vi "YJoint_Test.vi"() -> ()   [LabVIEW 2018]
uses:
  cluster_enum.ctl
  <vilib>/Utility/error.llb/DialogType.ctl
  <vilib>/DAQmx/read.llb/DAQmx Read (Analog 1D Wfm NChan NSamp).vi
  <vilib>/Waveform/WDTOps.llb/WDT Get Waveform Time Array DBL.vi
  <vilib>/DAQmx/configure/timing.llb/DAQmx Timing (Sample Clock).vi
  <vilib>/DAQmx/miscellaneous.llb/DAQmx Fill In Error Info.vi
  <resource>/objmgr/daqmx.rc
panel:
  out "Accel Card":waveform(dbl)[](graph) caption="Waveform Chart"
  in  "Tab Control":enum32{"Telemetry", "DAQ Settings"}(tab)
  in  "Accel Tare":bool caption="Reset"
  in  "Strain Card 1 Tare":bool caption="Reset"
  in  "Stop 4":bool caption="Stop"
  out "Save Path":path caption="Path"
  in  "Test Name":string caption="String"
  in  "Save 2":bool caption="Save"
  out "Accel Card Rate":dbl caption="Numeric"
  in  "Accel Card Sample Rate Setpoint":dbl=100.0 caption="Numeric"
  in  "Accel Card 1 Samples Per Loop":i32=100 caption="Numeric"
  in  "Strain Card 1 Rate Setpoint":dbl=1000.0 caption="Numeric"
  out "Strain Card 1 Rate":dbl caption="Numeric"
  in  "Strain Card 1 Samples Per Loop":i32=100 caption="Numeric"
  out "Strain Card 1":waveform(dbl)[](graph) caption="Waveform Chart"
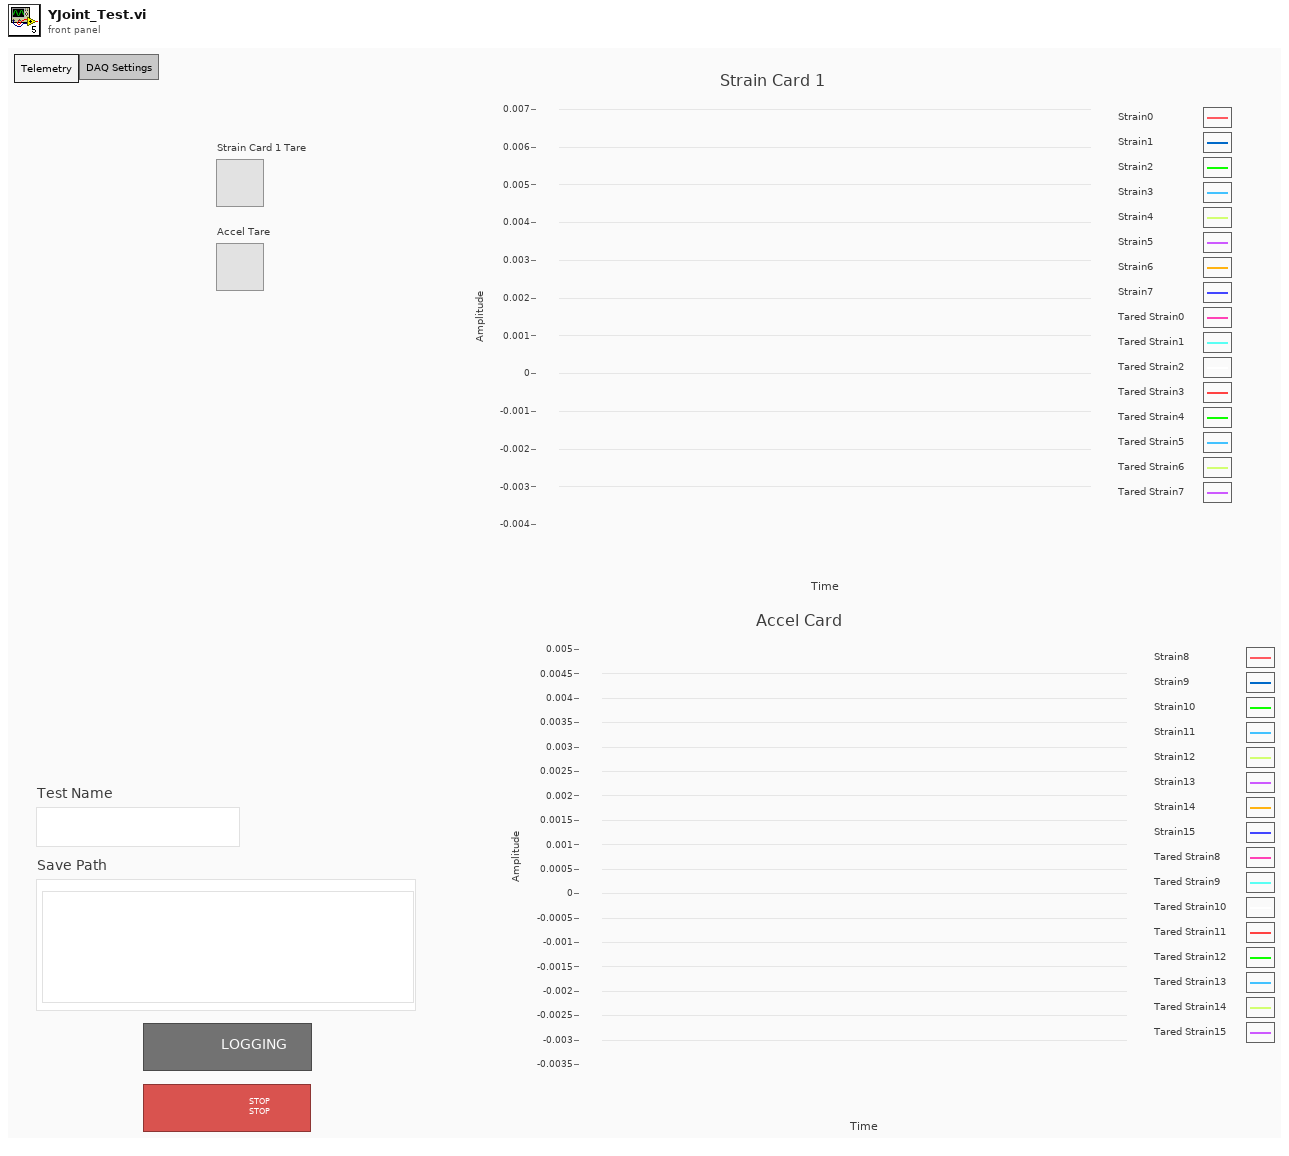
[diagram p1: front panel]
types:
  T1 = typedef "DialogType.ctl" = u16
  T2 = enum16{"open", "open or create", "create or replace", "create", "open (read-only)"}
  T3 = typedef "cluster_enum.ctl" = enum16{"Strain Card 2", "Strain Card 2 Tared", "Strain Card 1 Tared", "Strain Card 1", "Accel Card 1", "Accel Card 1 Tared", ""}
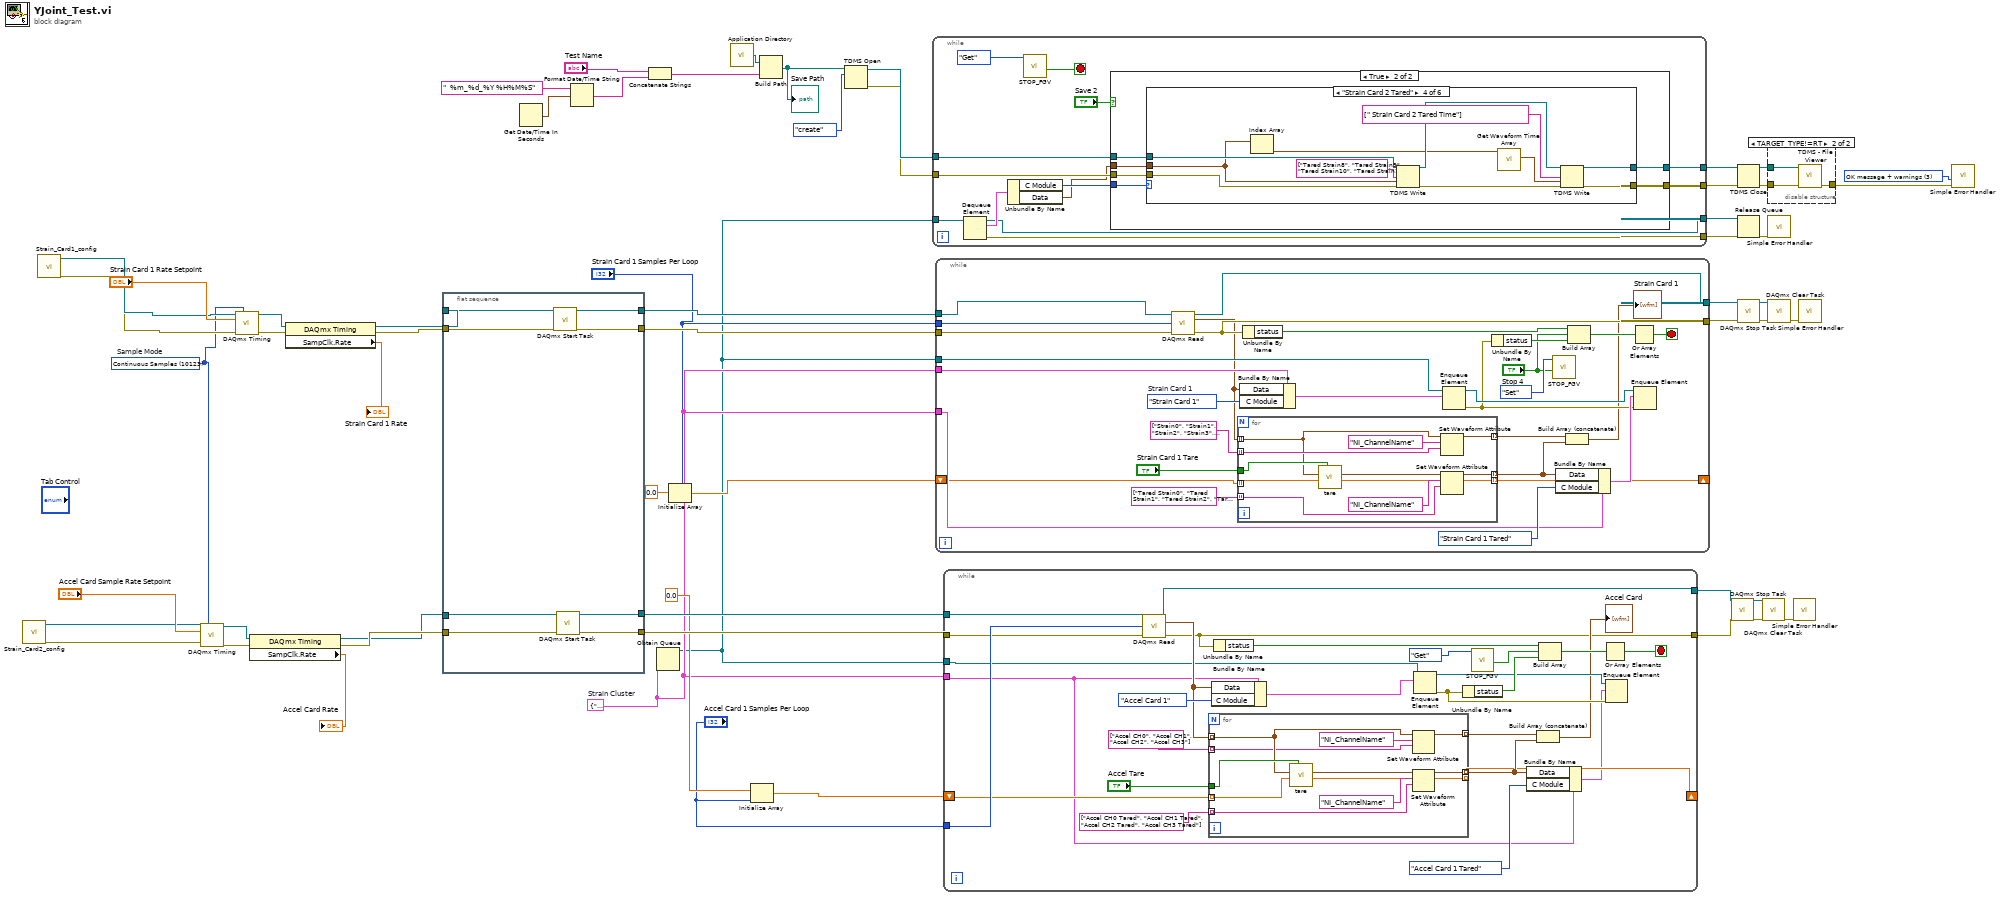
[diagram p0: block diagram]
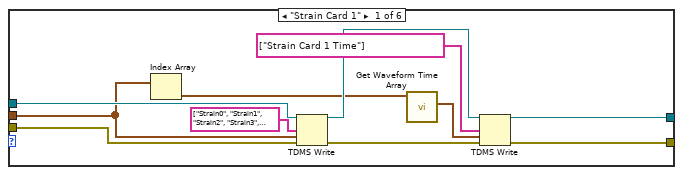
[diagram p4: hidden frame]
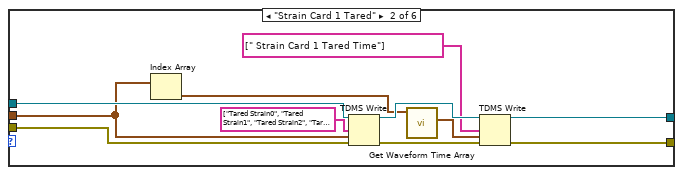
[diagram p5: hidden frame]
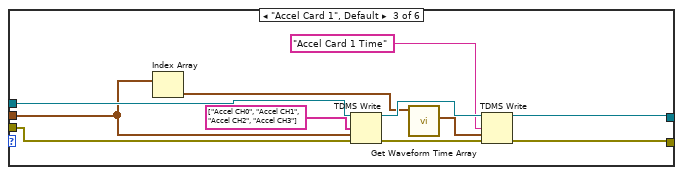
[diagram p6: hidden frame]
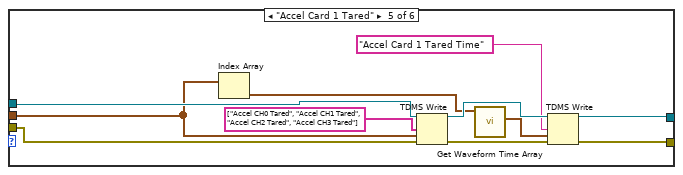
[diagram p7: hidden frame]
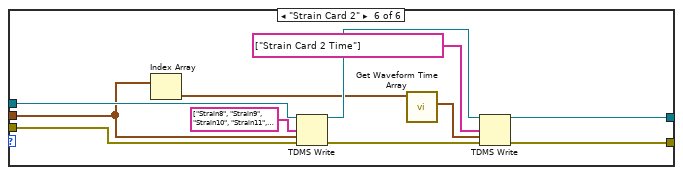
[diagram p8: hidden frame]
diagram:
  w35 = T1 3 items=["no dialog", "OK message", "continue or stop message", "OK message + warnings", "continue/stop + warnings"] ("type of dialog (OK msg:1)")
  w8 = cluster{"C Module":T3, " Data":waveform(dbl)[]} {"C Module"=enum."Strain Card 2", " Data"=[]}  # Strain Cluster
  w1 = 10123 items=["Finite Samples"=10178, "Continuous Samples"=10123, "Hardware Timed Single Point"=12522]  # Sample Mode
  n1 = call "Strain_Card2_config.vi"() -> ("error out"=w16:errorcluster, "task out"=w17:refnum<k21>)  [unwired: 10 in]
  n2 = call "Strain_Card1_config.vi"() -> ("error out"=w22:errorcluster, "task out"=w23:refnum<k21>)  [unwired: 10 in]
  n3 = call-poly <vilib>:"DAQmx Timing.vi"("task/channels in"=w17, "sample mode"=w1, "rate"="Accel Card Sample Rate Setpoint", "error in"=w16) -> ("task out"=w21:refnum<k21>, "error out"=w20:errorcluster)  [unwired: 10 in]
  n4 = call-poly <vilib>:"DAQmx Timing.vi"("task/channels in"=w23, "sample mode"=w1, "rate"="Strain Card 1 Rate Setpoint", "error in"=w22) -> ("task out"=w58:refnum<k21>, "error out"=w57:errorcluster)  [unwired: 10 in]
  n5 = property class="DAQmx Timing"(reference=w21, error in=w20) -> (reference out=w14:refnum<k21>, error out=w15:errorcluster, "SampClk.Rate"=→"Accel Card Rate":dbl)
  n6 = property class="DAQmx Timing"(reference=w58, error in=w57) -> (reference out=w56:refnum<k21>, error out=w55:errorcluster, "SampClk.Rate"=→"Strain Card 1 Rate":dbl)
  n7 = flat-sequence {
    tunnel: [w66] -> w52
    tunnel: w56 -> [w65]
    tunnel: w55 -> [w64]
    tunnel: [w63] -> w51
    tunnel: w15 -> [w62]
    tunnel: w14 -> [w61]
    tunnel: [w60] -> w13
    tunnel: [w59] -> w12
    frame #0 {
      n8 = call <vilib>:"DAQmx Start Task.vi"("task/channels in"=w65, "error in"=w64) -> ("task out"=w66:refnum<k21>, "error out"=w63:errorcluster)  [unwired: 12 in]
      n9 = call <vilib>:"DAQmx Start Task.vi"("task/channels in"=w61, "error in"=w62) -> ("task out"=w60:refnum<k21>, "error out"=w59:errorcluster)  [unwired: 12 in]
    }
  }
  n10 = Get Date/Time In Seconds() -> (seconds since 1Jan1904=w44:timestamp)
  n11 = Format Date/Time String(time format string (%c)="  %m_%d_%Y %H%M%S", seconds (now)=w44) -> (date/time string=w41:string)  [unwired: 1 in]
  n12 = Concatenate Strings("Test Name", w41) -> (w40:string)
  n13 = Obtain Queue(element data type=w8) -> (queue out=w7:refnum<queue>)  [unwired: 4 in, 2 out]
  n14 = Initialize Array(0.0 ("element"), "Strain Card 1 Samples Per Loop") -> (w24:dbl[])
  n15 = call <vilib>:"Application Directory.vi"() -> ("Application Directory"=w42:path)
  n16 = Initialize Array(0.0 ("element"), "Accel Card 1 Samples Per Loop") -> (w9:dbl[])
  n17 = Build Path(base path=w42, name or relative path=w40) -> (appended path=w39:path)
  "Save Path" <- w39
  n18 = TDMS Open(10:T2."create" ("operation"), 11:w39) -> (0:w36:errorcluster, 3:w37:refnum<k34>)  [unwired: 5 in]
  n19 = while {
    tunnel: w7 -> [w79]
    tunnel: w37 -> [w76]
    tunnel: w36 -> [w75]
    tunnel: [w73] -> w31
    tunnel: [w72] -> w30
    tunnel: [w68] -> w28
    tunnel: [w67] -> w27
    stop <- w70 stop-if-true
    n20 = Dequeue Element(queue=w79) -> (queue out=w68:refnum<queue>, element=w78:cluster{"C Module":T3, " Data":waveform(dbl)[]}, error out=w67:errorcluster)  [unwired: 2 in, 1 out]
    n21 = Unbundle By Name(w78) -> ("C Module"=w77:T3, "Data"=w74:waveform(dbl)[])
    n22 = call "STOP_FGV.vi"("Mode"=enum16{"Set", "Get"}."Get") -> ("Get Value"=w70:bool)  [unwired: 9 in, 1 out]
    n23 = case shown="True" "Save 2" {
      tunnel: w77 -> [_ w87]
      tunnel: w76 -> [w81 w86]
      tunnel: w75 -> [w80 w85]
      tunnel: w74 -> [_ w84]
      tunnel: [w81 w83] -> w73
      tunnel: [w80 w82] -> w72
      frame False {
      }
      frame True {
        n24 = case shown="\"Strain Card 2 Tared\"" w87 {
          tunnel: w86 -> [w98 w109 w114 w131 w135 w153]
          tunnel: w85 -> [w97 w108 w113 w130 w136 w152]
          tunnel: w84 -> [w91 w102 w112 w124 w134 w146]
          tunnel: [w93 w104 w111 w126 w138 w148] -> w83
          tunnel: [w94 w105 w110 w127 w137 w149] -> w82
          frame "Strain Card 1" {
            n25 = Index Array(array=w91) -> (element=w90:waveform(dbl))  [unwired: 1 in]
            n26 = TDMS Write(0:w98, 7:string[] ["Strain0", "Strain1", "Strain2", "Strain3", "Strain4", "Strain5", "Strain6", "Strain7"] ("channel name(s) in (Untitled)"), 9:w91, 11:w97) -> (4:w96:refnum<k34>, 15:w95:errorcluster)  [unwired: 2 in, 2 out]
            n27 = call-poly <vilib>:"Get Waveform Time Array.vi"("waveform in"=w90) -> ("X array"=w89:timestamp[])  [unwired: 9 in, 1 out]
            n28 = TDMS Write(0:w96, 7:string[] ["Strain Card 1 Time"] ("channel name(s) in (Untitled)"), 9:w89, 11:w95) -> (4:w93:refnum<k34>, 15:w94:errorcluster)  [unwired: 2 in, 2 out]
          }
          frame "Strain Card 1 Tared" {
            n29 = Index Array(array=w102) -> (element=w101:waveform(dbl))  [unwired: 1 in]
            n30 = TDMS Write(0:w109, 7:string[] ["Tared Strain0", "Tared Strain1", "Tared Strain2", "Tared Strain3", "Tared Strain4", "Tared Strain5", "Tared Strain6", "Tared Strain7"] ("channel name(s) in (Untitled)"), 9:w102, 11:w108) -> (4:w107:refnum<k34>, 15:w106:errorcluster)  [unwired: 2 in, 2 out]
            n31 = call-poly <vilib>:"Get Waveform Time Array.vi"("waveform in"=w101) -> ("X array"=w100:timestamp[])  [unwired: 9 in, 1 out]
            n32 = TDMS Write(0:w107, 7:string[] [" Strain Card 1 Tared Time"] ("channel name(s) in (Untitled)"), 9:w100, 11:w106) -> (4:w104:refnum<k34>, 15:w105:errorcluster)  [unwired: 2 in, 2 out]
          }
          frame "Accel Card 1", Default {
            n33 = Index Array(array=w112) -> (element=w118:waveform(dbl))  [unwired: 1 in]
            n34 = TDMS Write(0:w114, 7:string[] ["Accel CH0", "Accel CH1", "Accel CH2", "Accel CH3"] ("channel name(s) in (Untitled)"), 9:w112, 11:w113) -> (4:w120:refnum<k34>, 15:w119:errorcluster)  [unwired: 2 in, 2 out]
            n35 = call-poly <vilib>:"Get Waveform Time Array.vi"("waveform in"=w118) -> ("X array"=w117:timestamp[])  [unwired: 9 in, 1 out]
            n36 = TDMS Write(0:w120, 7:"Accel Card 1 Time", 9:w117, 11:w119) -> (4:w111:refnum<k34>, 15:w110:errorcluster)  [unwired: 2 in, 2 out]
          }
          frame "Strain Card 2 Tared" {
            n37 = Index Array(array=w124) -> (element=w123:waveform(dbl))  [unwired: 1 in]
            n38 = TDMS Write(0:w131, 7:string[] ["Tared Strain8", "Tared Strain9", "Tared Strain10", "Tared Strain11", "Tared Strain12", "Tared Strain13", "Tared Strain14", "Tared Strain15"] ("channel name(s) in (Untitled)"), 9:w124, 11:w130) -> (4:w129:refnum<k34>, 15:w128:errorcluster)  [unwired: 2 in, 2 out]
            n39 = call-poly <vilib>:"Get Waveform Time Array.vi"("waveform in"=w123) -> ("X array"=w122:timestamp[])  [unwired: 9 in, 1 out]
            n40 = TDMS Write(0:w129, 7:string[] [" Strain Card 2 Tared Time"] ("channel name(s) in (Untitled)"), 9:w122, 11:w128) -> (4:w126:refnum<k34>, 15:w127:errorcluster)  [unwired: 2 in, 2 out]
          }
          frame "Accel Card 1 Tared" {
            n41 = Index Array(array=w134) -> (element=w140:waveform(dbl))  [unwired: 1 in]
            n42 = TDMS Write(0:w135, 7:string[] ["Accel CH0 Tared", "Accel CH1 Tared", "Accel CH2 Tared", "Accel CH3 Tared"] ("channel name(s) in (Untitled)"), 9:w134, 11:w136) -> (4:w142:refnum<k34>, 15:w141:errorcluster)  [unwired: 2 in, 2 out]
            n43 = call-poly <vilib>:"Get Waveform Time Array.vi"("waveform in"=w140) -> ("X array"=w139:timestamp[])  [unwired: 9 in, 1 out]
            n44 = TDMS Write(0:w142, 7:"Accel Card 1 Tared Time", 9:w139, 11:w141) -> (4:w138:refnum<k34>, 15:w137:errorcluster)  [unwired: 2 in, 2 out]
          }
          frame "Strain Card 2" {
            n45 = Index Array(array=w146) -> (element=w145:waveform(dbl))  [unwired: 1 in]
            n46 = TDMS Write(0:w153, 7:string[] ["Strain8", "Strain9", "Strain10", "Strain11", "Strain12", "Strain13", "Strain14", "Strain15"] ("channel name(s) in (Untitled)"), 9:w146, 11:w152) -> (4:w151:refnum<k34>, 15:w150:errorcluster)  [unwired: 2 in, 2 out]
            n47 = call-poly <vilib>:"Get Waveform Time Array.vi"("waveform in"=w145) -> ("X array"=w144:timestamp[])  [unwired: 9 in, 1 out]
            n48 = TDMS Write(0:w151, 7:string[] ["Strain Card 2 Time"] ("channel name(s) in (Untitled)"), 9:w144, 11:w150) -> (4:w148:refnum<k34>, 15:w149:errorcluster)  [unwired: 2 in, 2 out]
          }
        }
      }
    }
  }
  n49 = while {
    tunnel: w52 -> [w178]
    tunnel: [w182] -> w48
    tunnel: w51 -> [w177]
    tunnel: [w175] -> w47
    tunnel: w7 -> [w171]
    tunnel: w8 -> [w174]
    tunnel: w8 -> [w168]
    tunnel: "Strain Card 1 Samples Per Loop" -> [w156]
    shift-right: [w154] -> _
    shift-left: w24 -> [w155]
    stop <- w181 stop-if-true
    w173 = cluster_enum."Strain Card 1"  # Strain Card 1
    n50 = call-poly <vilib>:"DAQmx Read.vi"("task/channels in"=w178, "number of samples per channel"=w156, "error in"=w177) -> ("task out"=w182:refnum<k21>, "data"=w161:waveform(dbl)[], "error out"=w175:errorcluster)  [unwired: 10 in]
    n51 = for {
      tunnel: w161 -> [w190] mode=indexing
      tunnel: [w185] -> w162 mode=indexing
      tunnel: "Strain Card 1 Tare" -> [w193]
      tunnel: string[] ["Strain0", "Strain1", "Strain2", "Strain3", "Strain4", "Strain5", "Strain6", "Strain7"] ("channel name(s) in (Untitled)") -> [w191] mode=indexing
      tunnel: [w189] -> w158 mode=indexing
      tunnel: string[] ["Tared Strain0", "Tared Strain1", "Tared Strain2", "Tared Strain3", "Tared Strain4", "Tared Strain5", "Tared Strain6", "Tared Strain7"] ("channel name(s) in (Untitled)") -> [w186] mode=indexing
      tunnel: w155 -> [w184] mode=indexing
      tunnel: [w183] -> w154 mode=indexing
      n52 = call "tare.vi"("Tare Control"=w193, "Shift Registor"=w184, "Input Waveform"=w190) -> ("Shift Registor Out"=w183:dbl, "output waveform"=w188:waveform(dbl))  [unwired: 7 in]
      n53 = Set Waveform Attribute(5:w191, 6:"NI_ChannelName" ("name"), 7:w190) -> (3:w189:waveform(dbl))  [unwired: 1 in, 2 out]
      n54 = Set Waveform Attribute(5:w186, 6:"NI_ChannelName" ("name"), 7:w188) -> (3:w185:waveform(dbl))  [unwired: 1 in, 2 out]
    }
    n55 = Bundle By Name(cluster=w174, "Data"=w161, "C Module"=w173) -> (w172:cluster{"C Module":T3, " Data":waveform(dbl)[]})
    n56 = Unbundle By Name(w175) -> ("status"=w180:bool)
    n57 = Enqueue Element(queue=w171, element=w172) -> (queue out=w166:refnum<queue>, error out=w165:errorcluster)  [unwired: 2 in, 1 out]
    n58 = Unbundle By Name(w165) -> ("status"=w176:bool)
    n59 = call "STOP_FGV.vi"("Set Value"="Stop 4", "Mode"=enum16{"Set", "Get"}."Set") -> ()  [unwired: 8 in, 2 out]
    n60 = Bundle By Name(cluster=w168, "Data"=w162, "C Module"=cluster_enum."Strain Card 1 Tared" ("Strain Card 1")) -> (w167:cluster{"C Module":T3, " Data":waveform(dbl)[]})
    n61 = Build Array (concatenate)(w158, w162) -> (→"Strain Card 1":waveform(dbl)[])
    n62 = Build Array(w180, "Stop 4", w176) -> (w179:bool[])
    n63 = Or Array Elements(Boolean array=w179) -> (logical OR=w181:bool)
    n64 = Enqueue Element(queue=w166, element=w167, error in (no error)=w165) -> ()  [unwired: 1 in, 3 out]
  }
  n65 = while {
    tunnel: w13 -> [w205]
    tunnel: w12 -> [w203]
    tunnel: "Accel Card 1 Samples Per Loop" -> [w204]
    shift-right: [w198] -> _
    shift-left: w9 -> [w202]
    tunnel: w8 -> [w197]
    tunnel: w7 -> [w201]
    tunnel: [w200] -> w3
    tunnel: [w199] -> w2
    stop <- w196 stop-if-true
    n66 = call-poly <vilib>:"DAQmx Read.vi"("task/channels in"=w205, "number of samples per channel"=w204, "error in"=w203) -> ("task out"=w200:refnum<k21>, "data"=w210:waveform(dbl)[], "error out"=w199:errorcluster)  [unwired: 10 in]
    n67 = for {
      tunnel: w210 -> [w228] mode=indexing
      tunnel: [w231] -> w209 mode=indexing
      tunnel: "Accel Tare" -> [w232]
      tunnel: string[] ["Accel CH0 Tared", "Accel CH1 Tared", "Accel CH2 Tared", "Accel CH3 Tared"] ("channel name(s) in (Untitled)") -> [w226] mode=indexing
      tunnel: string[] ["Accel CH0", "Accel CH1", "Accel CH2", "Accel CH3"] ("channel name(s) in (Untitled)") -> [w225] mode=indexing
      tunnel: [w227] -> w206 mode=indexing
      tunnel: [w223] -> w198 mode=indexing
      tunnel: w202 -> [w222] mode=indexing
      n68 = call "tare.vi"("Tare Control"=w232, "Shift Registor"=w222, "Input Waveform"=w228) -> ("Shift Registor Out"=w223:dbl, "output waveform"=w230:waveform(dbl))  [unwired: 7 in]
      n69 = Set Waveform Attribute(5:w225, 6:"NI_ChannelName" ("name"), 7:w228) -> (3:w227:waveform(dbl))  [unwired: 1 in, 2 out]
      n70 = Set Waveform Attribute(5:w226, 6:"NI_ChannelName" ("name"), 7:w230) -> (3:w231:waveform(dbl))  [unwired: 1 in, 2 out]
    }
    n71 = Bundle By Name(cluster=w197, "Data"=w210, "C Module"=cluster_enum."Accel Card 1" ("Strain Card 1")) -> (w217:cluster{"C Module":T3, " Data":waveform(dbl)[]})
    n72 = Unbundle By Name(w199) -> ("status"=w221:bool)
    n73 = Enqueue Element(queue=w201, element=w217) -> (queue out=w215:refnum<queue>, error out=w214:errorcluster)  [unwired: 2 in, 1 out]
    n74 = Unbundle By Name(w214) -> ("status"=w219:bool)
    n75 = call "STOP_FGV.vi"("Mode"=enum16{"Set", "Get"}."Get") -> ("Get Value"=w211:bool)  [unwired: 9 in, 1 out]
    n76 = Bundle By Name(cluster=w197, "Data"=w209, "C Module"=cluster_enum."Accel Card 1 Tared" ("Strain Card 1")) -> (w195:cluster{"C Module":T3, " Data":waveform(dbl)[]})
    n77 = Build Array (concatenate)(w206, w209) -> (→"Accel Card":waveform(dbl)[])
    n78 = Build Array(w221, w211, w219) -> (w220:bool[])
    n79 = Or Array Elements(Boolean array=w220) -> (logical OR=w196:bool)
    n80 = Enqueue Element(queue=w215, element=w195, error in (no error)=w214) -> ()  [unwired: 1 in, 3 out]
  }
  n81 = call <vilib>:"DAQmx Stop Task.vi"("task/channels in"=w3, "error in"=w2) -> ("task out"=w6:refnum<k21>, "error out"=w5:errorcluster)  [unwired: 12 in]
  n82 = TDMS Close(8:w30, 11:w31) -> (0:w33:errorcluster, 3:w34:path)
  n83 = Release Queue(queue=w28, error in (no error)=w27) -> (error out=w29:errorcluster)  [unwired: 1 in, 2 out]
  n84 = call <vilib>:"DAQmx Stop Task.vi"("task/channels in"=w48, "error in"=w47) -> ("task out"=w50:refnum<k21>, "error out"=w49:errorcluster)  [unwired: 12 in]
  n85 = call <vilib>:"DAQmx Clear Task.vi"("task in"=w6, "error in"=w5) -> ("error out"=w4:errorcluster)  [unwired: 13 in]
  n86 = disable-structure shown="TARGET_TYPE!=RT" {
    disable-tunnel: w33 -> [w233 w236]
    disable-tunnel: w34 -> [_ w235]
    disable-tunnel: [w233 w234] -> w32
    frame condition #0 {
    }
    frame condition #1 (active) {
      n87 = call <vilib>:"TDMS - File Viewer.vi"("error in (no error)"=w236, "file path"=w235) -> ("error out"=w234:errorcluster)  [unwired: 5 out]
    }
  }
  n88 = call <vilib>:"Simple Error Handler.vi"("error in (no error)"=w29) -> ()  [unwired: 1 in, 8 out]
  n89 = call <vilib>:"DAQmx Clear Task.vi"("task in"=w50, "error in"=w49) -> ("error out"=w46:errorcluster)  [unwired: 13 in]
  n90 = call <vilib>:"Simple Error Handler.vi"("error in (no error)"=w4) -> ()  [unwired: 1 in, 8 out]
  n91 = call <vilib>:"Simple Error Handler.vi"("error in (no error)"=w46) -> ()  [unwired: 1 in, 8 out]
  n92 = call <vilib>:"Simple Error Handler.vi"("type of dialog (OK msg:1)"=w35, "error in (no error)"=w32) -> ()  [unwired: 1 in, 7 out]
